vi "Convert Termperature.vi"(1 "Raw Voltage":dbl) -> (0 "Temperature":dbl)   [LabVIEW 2016]
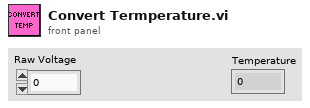
[diagram p1: front panel]
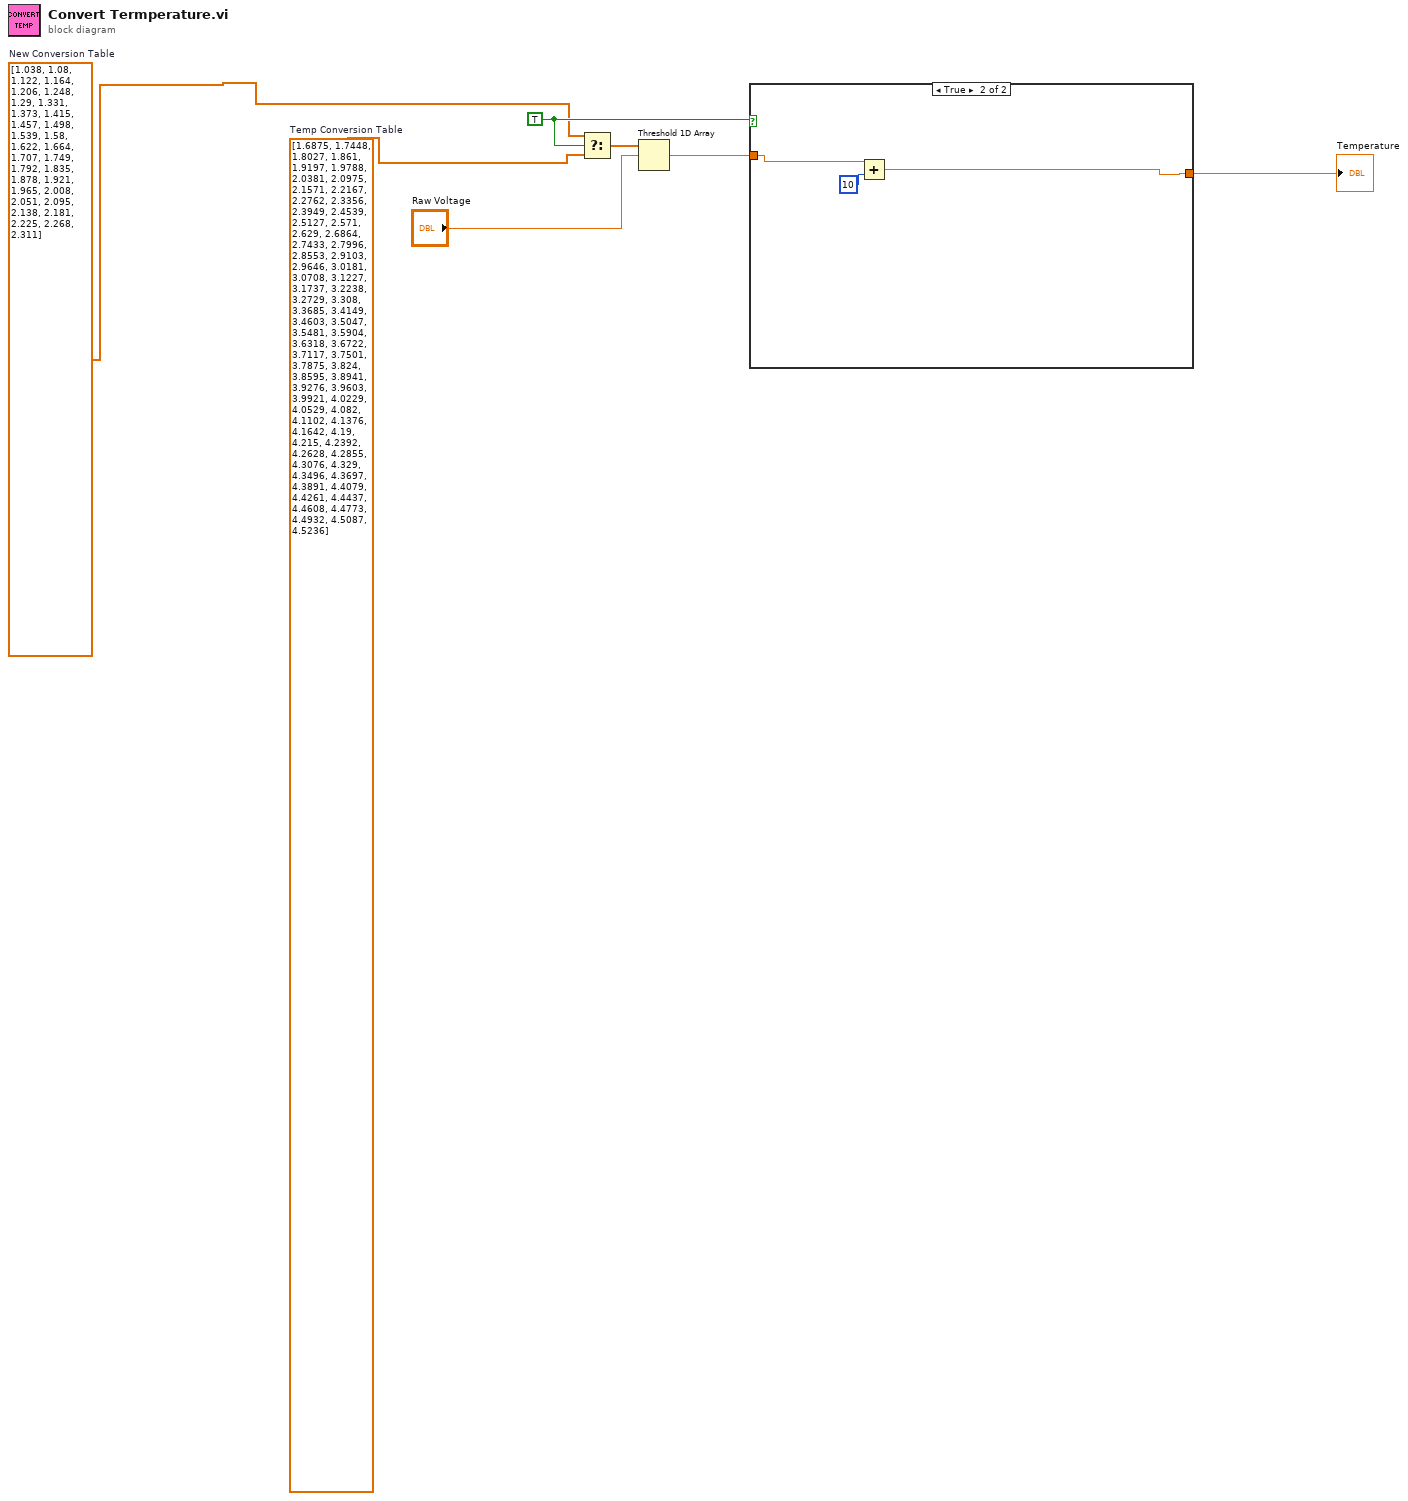
[diagram p0: block diagram]
diagram:
  w1 = dbl[] [1.038, 1.08, 1.122, 1.164, 1.206, 1.248, 1.29, 1.331, 1.373, 1.415, 1.457, 1.498, 1.539, 1.58, 1.622, 1.664, 1.707, 1.749, 1.792, 1.835, 1.878, 1.921, 1.965, 2.008, 2.051, 2.095, 2.138, 2.181, 2.225, 2.268, 2.311]  # New Conversion Table
  w4 = TRUE
  w6 = dbl[] [1.6875, 1.7448, 1.8027, 1.861, 1.9197, 1.9788, 2.0381, 2.0975, 2.1571, 2.2167, 2.2762, 2.3356, 2.3949, 2.4539, 2.5127, 2.571, 2.629, 2.6864, 2.7433, 2.7996, 2.8553, 2.9103, 2.9646, 3.0181, 3.0708, 3.1227, 3.1737, 3.2238, 3.2729, 3.308, 3.3685, 3.4149, 3.4603, 3.5047, 3.5481, 3.5904, 3.6318, 3.6722, 3.7117, 3.7501, 3.7875, 3.824, 3.8595, 3.8941, 3.9276, 3.9603, 3.9921, 4.0229, 4.0529, 4.082, 4.1102, 4.1376, 4.1642, 4.19, 4.215, 4.2392, 4.2628, 4.2855, 4.3076, 4.329, 4.3496, 4.3697, 4.3891, 4.4079, 4.4261, 4.4437, 4.4608, 4.4773, 4.4932, 4.5087, 4.5236]  # Temp Conversion Table
  n1 = Select(t=w1, s=w4, f=w6) -> (s? t:f=w5:dbl[])
  n2 = Threshold 1D Array(2:"Raw Voltage", 3:w5) -> (0:w3:dbl)  [unwired: 1 in]
  n3 = case shown="True" w4 {
    tunnel: w3 -> [w8 w9]
    tunnel: [w8 w10] -> w2
    frame False {
    }
    frame True {
      n4 = Add(x=w9, y=10) -> (x+y=w10:dbl)
    }
  }
  "Temperature" <- w2
